vi "Vision Processing.vi"(4 "error in (no error)":errorcluster) -> ()   [LabVIEW 2012]
doc: "This VI runs in parallel to other tasks. It gets images from the camera, processes them for color or shape and use that information to affect robot behavior."
uses:
  Robot Global Data.vi
  <vilib>/vision/NI_Vision_Development_Module.lvlib
panel:
  out "Position":cluster{"x":sgl, "y":sgl}
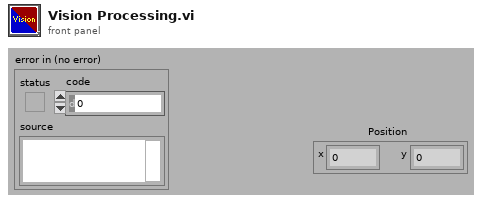
[diagram p1: front panel]
types:
  T1 = typedef "Image Type" = u32
  T2 = typedef "IMAQ Image.ctl" = refnum<image>
  T3 = typedef "WPI_CameraDevRef.ctl" = cluster{"Camera Address":string, "CameraStatus":errorcluster, "Acquire Image Notifier":refnum<notifier>}
  T4 = cluster{"Position":cluster{"x":sgl, "y":sgl}, "Angle":sgl, "Scale":sgl, "Score":sgl, "Bounding Box":cluster{"x":sgl, "y":sgl}[]}[]
  T5 = cluster{"Position":cluster{"x":sgl, "y":sgl}, "Angle":sgl, "Scale":sgl, "Score":sgl, "Bounding Box":cluster{"x":sgl, "y":sgl}[]}
  T6 = typedef "WPI_CameraImageSize.ctl" = enum16{"640x480", "320x240", "160x120"}
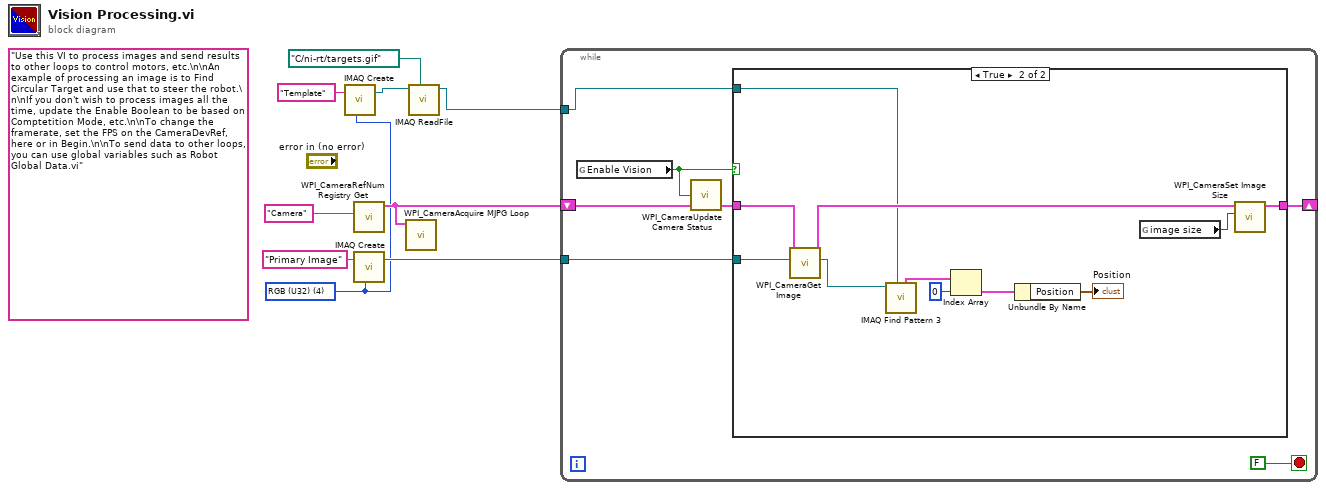
[diagram p0: block diagram]
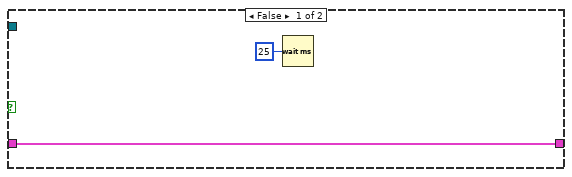
[diagram p2: hidden frame]
diagram:
  (unwired) "Use this VI to process images and send results to other loops to control motors, etc.\n\nAn example of processing an image is to Find Circular Target and use that to steer the robot.\n\nIf you don't wish to process images all the time, update the Enable Boolean to be based on Comptetition Mode, etc.\n\nTo change the framerate, set the FPS on the CameraDevRef, here or in Begin.\n\nTo send data to other loops, you can use global variables such as Robot Global Data.vi"
  w3 = T1 4 items=["Grayscale (U8)", "Grayscale (I16)", "Grayscale (SGL)", "Complex (CSG)", "RGB (U32)", "HSL (U32)", "RGB (U64)"] ("Image Type")
  n1 = call "IMAQ Create"("Image Name"="Template", "Image Type"=w3) -> ("New Image"=w5:T2)  [unwired: 3 in, 1 out]
  n2 = call <vilib>:"WPI_CameraRefNum Registry Get.vi"("refnum name"="Camera") -> ("CameraDevRef"=w6:T3)  [unwired: 1 in, 9 out]
  n3 = call "IMAQ Create"("Image Name"="Primary Image", "Image Type"=w3) -> ("New Image"=w8:T2)  [unwired: 2 in, 2 out]
  n4 = call <vilib>:"WPI_CameraAcquire MJPG Loop.vi"("CameraDevRef"=w6) -> ()  [unwired: 11 in]
  n5 = call "IMAQ ReadFile"("File Path"=path "C:/ni-rt/targets.gif", "Image"=w5) -> ("Image Out"=w1:T2)  [unwired: 5 in, 4 out]
  n6 = while {
    shift-right: [w15] -> _
    shift-left: w6 -> [w13]
    tunnel: w8 -> [w14]
    tunnel: w1 -> [w10]
    stop <- FALSE stop-if-true
    n7 = global read "Robot Global Data.vi" "Enable Vision"() -> (w11:bool)
    n8 = call <vilib>:"WPI_CameraUpdate Camera Status.vi"("CameraDevRef In"=w13, "Enable Vision"=w11) -> ("CameraDevRef Out"=w12:T3)  [unwired: 3 in]
    n9 = case shown="True" w11 {
      tunnel: w14 -> [_ w28]
      tunnel: [w18 w29] -> w15
      tunnel: w12 -> [w18 w26]
      tunnel: w10 -> [_ w24]
      frame False {
        n10 = Wait (ms)(milliseconds to wait=u32 25) -> ()  [unwired: 1 out]
      }
      frame True {
        n11 = call <vilib>:"WPI_CameraGet Image.vi"("Image"=w28, "CameraDevRef"=w26) -> ("Image Out"=w23:T2, "CameraDevRef Out"=w25:T3)  [unwired: 1 in, 7 out]
        n12 = call "IMAQ Find Pattern 3"("Template"=w24, "Image"=w23) -> ("Matches"=w22:T4)  [unwired: 4 in, 5 out]
        n13 = Index Array(array=w22, index=0) -> (element=w20:T5)
        n14 = Unbundle By Name(w20) -> ("Position"=→"Position":cluster{"x":sgl, "y":sgl})
        n15 = global read "Robot Global Data.vi" "image size"() -> (w27:T6)
        n16 = call <vilib>:"WPI_CameraSet Image Size.vi"("Image Size"=w27, "CameraDevRef"=w25) -> ("CameraDevRef Out"=w29:T3)  [unwired: 1 in, 8 out]
      }
    }
  }
